vi "WriteEmbedded.vi"(8 "error in (no error)":errorcluster, 10 "Subpanels":refnum<class "EmbeddedSMO.lvclass">[](array[class]), 11 "MAUI in":refnum<class "MAUI.lvclass">) -> (0 "error out":errorcluster, 3 "MAUI out":refnum<class "MAUI.lvclass">)   [LabVIEW 2016, in "MAUI.lvclass"]
uses:
  MAUI.lvclass
  <vilib>/Levylab/Embedded SMO UI/EmbeddedSMO.lvclass
  Typedefs/PrivateEvents--MAUI.SetEmbedded.ctl
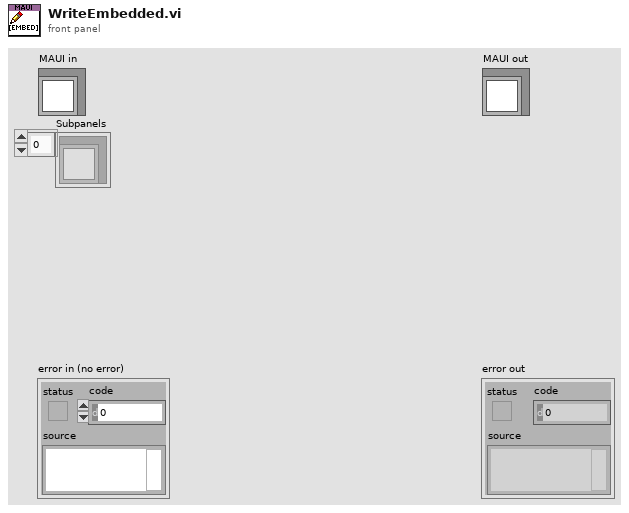
[diagram p1: front panel]
types:
  T1 = typedef "MAUI.lvclass/PrivateEvents--MAUI.SetEmbedded.ctl" = cluster{"Subpanels":refnum<class "EmbeddedSMO.lvclass">[]}
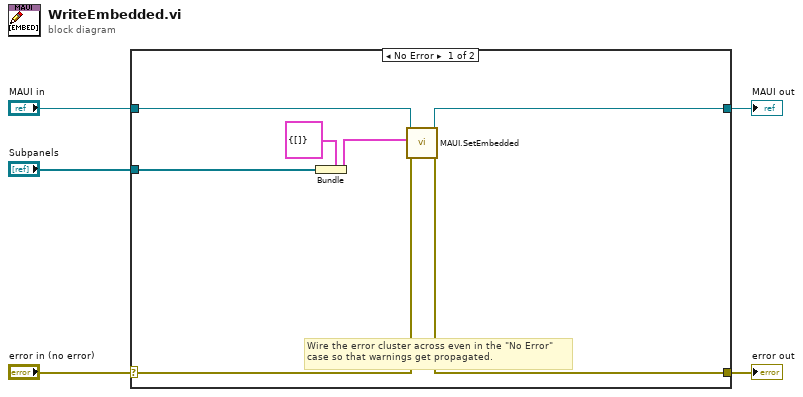
[diagram p0: block diagram]
diagram:
  n1 = case shown="No Error" "error in (no error)" {
    selector: "error in (no error)" -> [w10 w14]
    tunnel: [w9 w14] -> w4
    tunnel: [w11 w13] -> w2
    tunnel: "MAUI in" -> [w12 w13]
    tunnel: "Subpanels" -> [w7 _]
    frame No Error {
      # "Wire the error cluster across even in the \"No Error\"\ncase so that warnings get propagated."
      n2 = Bundle(cluster=T1 {"Subpanels"=[]} ("SetEmbedded"), "Subpanels"=w7) -> (w6:T1)
      n3 = call "MAUI.SetEmbedded.vi"("error in (no error)"=w10, "SetEmbedded"=w6, "MAUI"=w12) -> ("error out"=w9:errorcluster, "MAUI out"=w11:refnum<class "MAUI.lvclass">)  [unwired: 7 in]
    }
    frame Error {
    }
  }
  "error out" <- w4
  "MAUI out" <- w2
